vi "Populate Voltage Scaling FPGA Data.vi"(6 "DataReplayVoltages in":T1[](array[typedef]), 8 "error in (no error)":errorcluster, 11 "FPGA Interface Base in":refnum<class "FPGA Interface Base.lvclass">) -> (0 "error out":errorcluster, 3 "FPGA Interface Base out":refnum<class "FPGA Interface Base.lvclass">, 4 "DataReplayVoltages out":T1[](array[typedef]))   [LabVIEW 2011, in "Engine Sim RT.lvlib"]
uses:
  Engine Sim RT.lvlib
  <userlib>/_FPGA Interface Advanced Tools/FPGA Interface Base/FPGA Interface Base.lvclass
  Shared/DataReplayVoltageConfig.ctl
  <vilib>/rvi/DataTransferAndStorage/Container/Common/niFpgaDataTypeControl.ctl
  <userlib>/_FPGA Interface Advanced Tools/FPGA Interface Base/FPGA Interface Base.lvclass/FPGA Interface Base.ctl
  <vilib>/Utility/error.llb/Error Cluster From Error Code.vi
  Engine Simulation Shared.lvlib
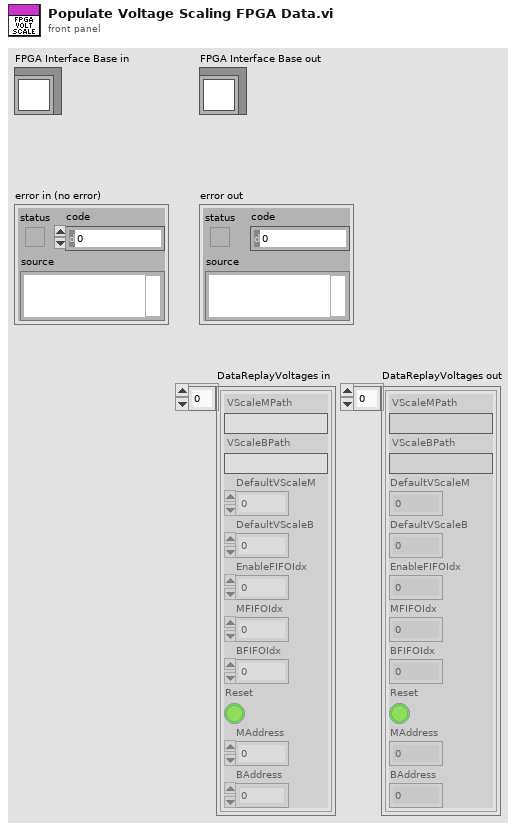
[diagram p1: front panel]
types:
  T1 = typedef "Engine Simulation Shared.lvlib/DataReplayVoltageConfig.ctl" = cluster{"VScaleMPath":string, "VScaleBPath":string, "DefaultVScaleM":u32, "DefaultVScaleB":i32, "EnableFIFOIdx":i32, "MFIFOIdx":i32, "BFIFOIdx":i32, "Reset":bool, "MAddress":u32, "BAddress":u32}
  T2 = typedef "niFpgaDataTypeControl.ctl" = enum32{"Boolean", "I8", "I16", "I32", "I64", "U8", "U16", "U32", "U64", "FXP", "CustomControl"}
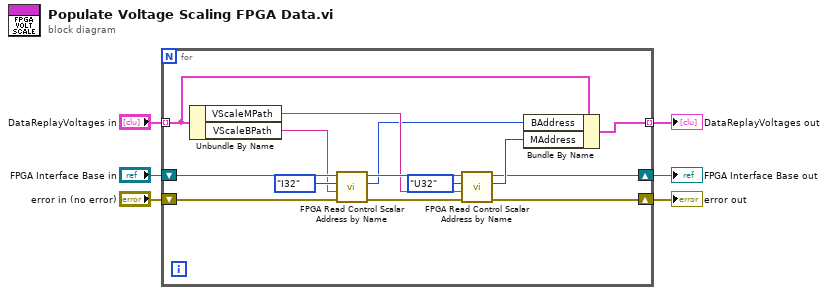
[diagram p0: block diagram]
diagram:
  n1 = for {
    shift-right: [w9] -> w1
    shift-left: "error in (no error)" -> [w20]
    shift-right: [w8] -> w3
    shift-left: "FPGA Interface Base in" -> [w19]
    tunnel: "DataReplayVoltages in" -> [w12] mode=indexing
    tunnel: [w7] -> w2 mode=indexing
    n2 = Unbundle By Name(w12) -> ("VScaleMPath"=w13:string, "VScaleBPath"=w17:string)
    n3 = call <userlib>:"FPGA Read Control Scalar Address by Name.vi"("error in (no error)"=w20, "Name"=w17, "Data Type"=niFpgaDataTypeControl."I32", "FPGA Interface Base in"=w19) -> ("error out"=w16:errorcluster, "Address"=w11:u32, "FPGA Interface Base out"=w15:refnum<class "FPGA Interface Base.lvclass">)  [unwired: 4 in, 1 out]
    n4 = call <userlib>:"FPGA Read Control Scalar Address by Name.vi"("error in (no error)"=w16, "Name"=w13, "Data Type"=niFpgaDataTypeControl."U32", "FPGA Interface Base in"=w15) -> ("error out"=w9:errorcluster, "Address"=w10:u32, "FPGA Interface Base out"=w8:refnum<class "FPGA Interface Base.lvclass">)  [unwired: 4 in, 1 out]
    n5 = Bundle By Name(cluster=w12, "BAddress"=w11, "MAddress"=w10) -> (w7:T1)
  }
  "FPGA Interface Base out" <- w3
  "error out" <- w1
  "DataReplayVoltages out" <- w2
